vi "Create Measurement Plugin SubVIs - Multiple Converter.vi"(11 "error in":errorcluster) -> (15 "error out":errorcluster)   [LabVIEW 2021, in "Converter.lvlib"]
uses:
  Converter.lvlib
  Path Functions/Path Functions.lvlib
  Converter Reusables/Converter Reusables.lvlib
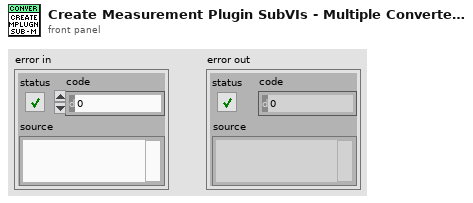
[diagram p1: front panel]
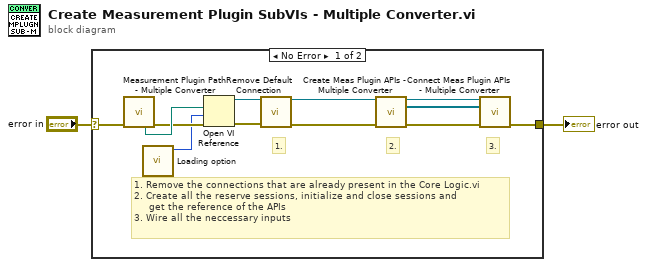
[diagram p0: block diagram]
diagram:
  n1 = case shown="No Error" "error in" {
    selector: "error in" -> [w11 w15]
    tunnel: [w6 w15] -> w2
    frame No Error {
      # "1. Remove the connections that are already present in the Core Logic.vi\n2. Create all the reserve sessions, initialize and close sessions and\n     get the reference of the APIs\n3. Wire all the neccessary inputs"
      # "3."
      # "2."
      # "1."
      n2 = call "Measurement Plugin Path - Multiple Converter.vi"("error in"=w11) -> ("logic vi path"=w12:path, "error out"=w10:errorcluster)  [unwired: 2 in, 11 out]
      n3 = call "Loading option.vi"() -> ("options"=w3:i32)  [unwired: 11 in]
      n4 = Open VI Reference(vi path=w12, options=w3, error in (no error)=w10) -> (vi reference=w14:refnum<vi>, error out=w13:errorcluster)  [unwired: 3 in]
      n5 = call "Remove Default Connection.vi"("vi reference"=w14, "error in"=w13) -> ("vi reference out"=w8:refnum<vi>, "error out"=w9:errorcluster)  [unwired: 12 in]
      n6 = call "Create Meas Plugin APIs - Multiple Converter.vi"("logic vi in"=w8, "error in"=w9) -> ("logic vi out"=w5:refnum<vi>, "sub vi refrences"=w4:refnum<vi>[], "error out"=w7:errorcluster)  [unwired: 11 in]
      n7 = call "Connect Meas Plugin APIs - Multiple Converter.vi"("logic vi ref"=w5, "sub vis"=w4, "error in"=w7) -> ("error out"=w6:errorcluster)  [unwired: 12 in]
    }
    frame Error {
    }
  }
  "error out" <- w2
